vi "exercicios3_numeric.vi"() -> ()   [LabVIEW 2018]
panel:
  out "32bit integer":i32
  out "Somatório Total":dbl
  out "x+y 2":dbl
  out "x/y":dbl
  out "Área":dbl
  out "Perda de Carga Localizada":dbl
  out "x+y":dbl
  in  "y":dbl
  in  "x":dbl
  # "Soma"
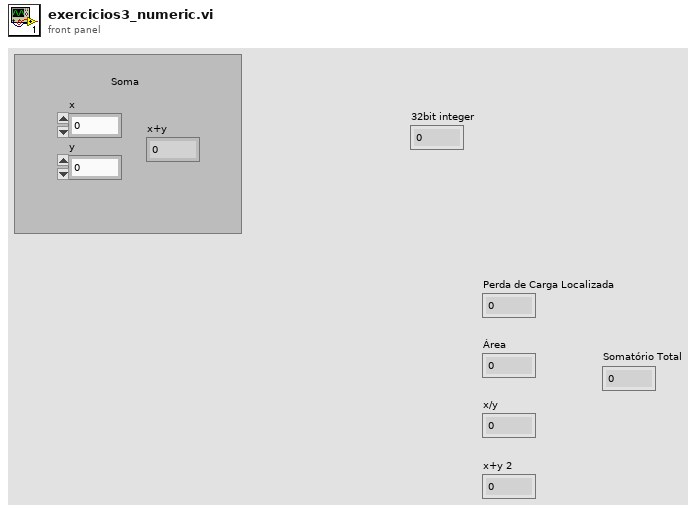
[diagram p1: front panel]
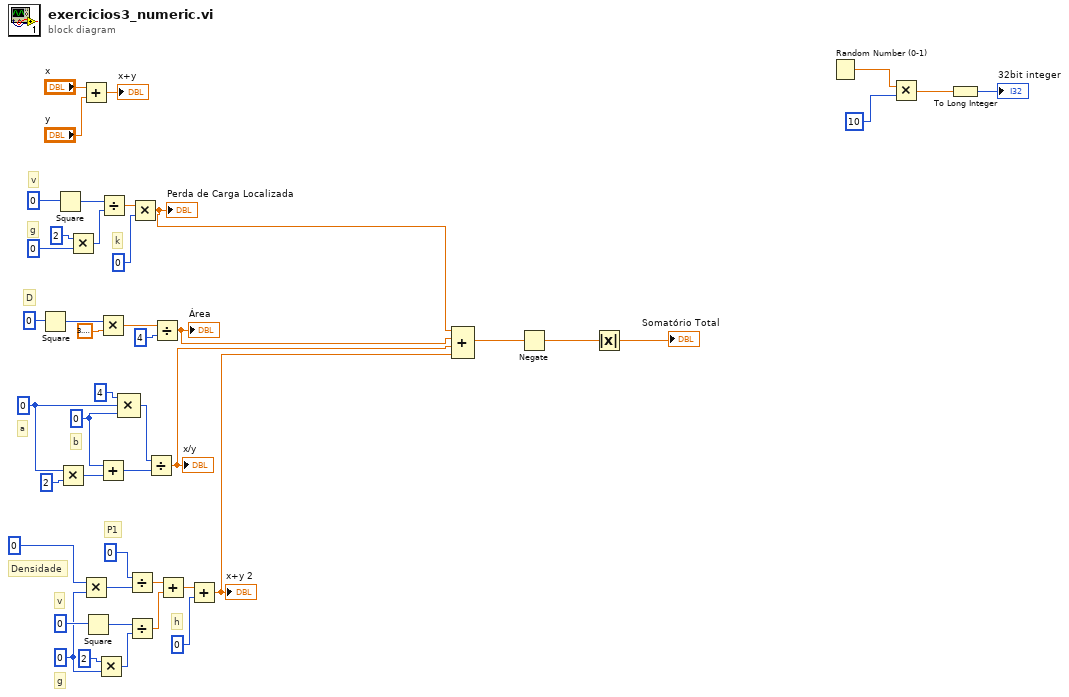
[diagram p0: block diagram]
diagram:
  w15 = 0
  w25 = 0
  w27 = 0
  # "h"
  # "v"
  # "g"
  # "Densidade"
  # "P1"
  # "b"
  # "a"
  # "D"
  # "g"
  # "v"
  # "k"
  n1 = Square(x=0) -> (x^2=w34:i32)
  n2 = Square(x=0) -> (x^2=w42:i32)
  n3 = Multiply(x=w27, y=2) -> (x*y=w26:i32)
  n4 = Multiply(x=2, y=0) -> (x*y=w39:i32)
  n5 = Add(x="x", y="y") -> (x+y=→"x+y":dbl)
  n6 = Multiply(x=0, y=w15) -> (x*y=w21:i32)
  n7 = Square(x=0) -> (x^2=w18:i32)
  n8 = Multiply(x=2, y=w15) -> (x*y=w16:i32)
  n9 = Multiply(x=w34, y=3.141592653589793) -> (x*y=w32:dbl)
  n10 = Add(x=w25, y=w26) -> (x+y=w24:i32)
  n11 = Divide(x=w42, y=w39) -> (x/y=w38:dbl)
  n12 = Compound Arithmetic op=MULTIPLY(4, w27, w25) -> (w29:i32)
  n13 = Divide(x=0, y=w21) -> (x/y=w20:dbl)
  n14 = Divide(x=w18, y=w16) -> (x/y=w14:dbl)
  n15 = Multiply(x=w38, y=0) -> (x*y=w11:dbl)
  "Perda de Carga Localizada" <- w11
  n16 = Divide(x=w29, y=w24) -> (x/y=w9:dbl)
  "x/y" <- w9
  n17 = Divide(x=w32, y=4) -> (x/y=w10:dbl)
  "Área" <- w10
  n18 = Add(x=w20, y=w14) -> (x+y=w13:dbl)
  n19 = Add(x=w13, y=0) -> (x+y=w8:dbl)
  "x+y 2" <- w8
  n20 = Compound Arithmetic op=unknown(w11, w10, w9, w8) -> (w7:dbl)
  n21 = Negate(x=w7) -> (-x=w6:dbl)
  n22 = Absolute Value(x=w6) -> (abs(x)=→"Somatório Total":dbl)
  n23 = Random Number (0-1)() -> (number: 0 to 1=w4:dbl)
  n24 = Multiply(x=w4, y=10) -> (x*y=w2:dbl)
  n25 = To Long Integer(number=w2) -> (32bit integer=→"32bit integer":i32)
